vi "extract reports.vi"() -> ()   [LabVIEW 2013]
panel:
  out "error out":errorcluster
  in  "Op":T1(ring)
  out "text":string[](array[string])
  in  "error in":errorcluster
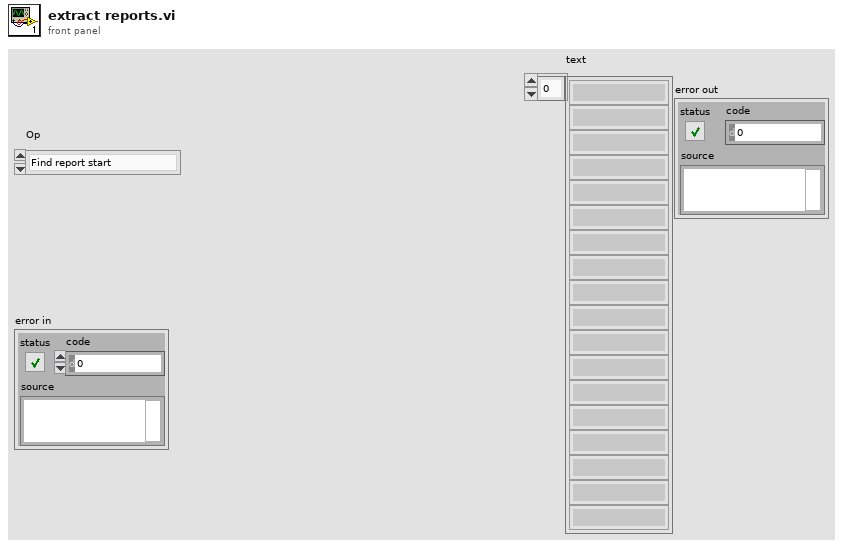
[diagram p1: front panel]
types:
  T1 = enum16{"Find report start", "Collect report body", "Find report end"}
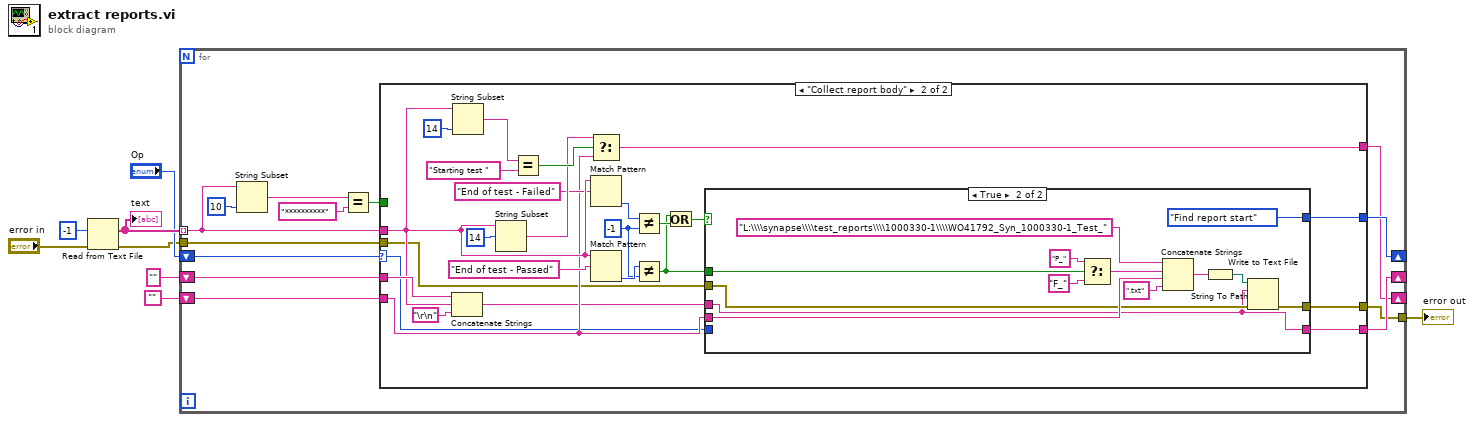
[diagram p0: block diagram]
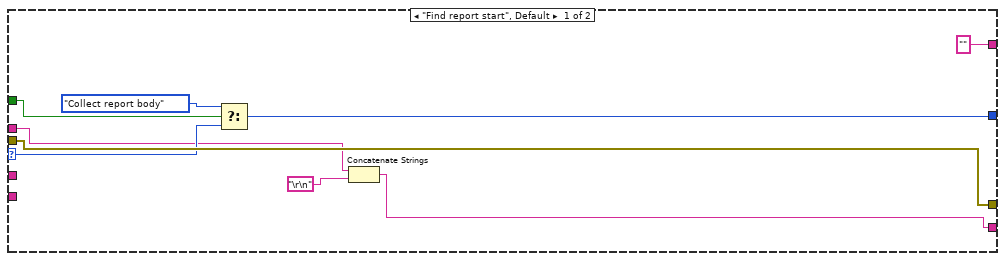
[diagram p2: hidden frame]
diagram:
  n1 = Read from Text File(count=-1, error in="error in") -> (text=w6:string[], error out=w2:errorcluster)  [unwired: 2 in, 2 out]
  "text" <- w6
  n2 = for {
    tunnel: w6 -> [w17] mode=indexing
    shift-right: [w14] -> _
    shift-left: "" -> [w16]
    shift-right: [w13] -> _
    shift-left: "Op" -> [w15]
    shift-right: [w11] -> _
    shift-left: "" -> [w12]
    tunnel: w2 -> [w10]
    tunnel: [w9] -> w1
    n3 = String Subset(string=w17, length (rest)=10 ("length (rest)")) -> (substring=w20:string)  [unwired: 1 in]
    n4 = Equal?(x=w20, y="**********") -> (x = y?=w18:bool)
    n5 = case shown="\"Collect report body\"" w15 {
      selector: w15 -> [w27 w34]
      tunnel: w18 -> [w29 _]
      tunnel: w17 -> [w24 w46]
      tunnel: w16 -> [_ w55]
      tunnel: [w22 w31] -> w14
      tunnel: [w26 w33] -> w13
      tunnel: w12 -> [_ w38]
      tunnel: ["" w48] -> w11
      tunnel: w10 -> [w30 w36]
      tunnel: [w30 w35] -> w9
      frame "Find report start", Default {
        n6 = Select(t=T1."Collect report body" ("Op"), s=w29, f=w27) -> (s? t:f=w26:T1)
        n7 = Concatenate Strings(w24, "\r\n") -> (w22:string)
      }
      frame "Collect report body" {
        w42 = -1 ("y")
        n8 = Concatenate Strings(w55, w46, "\r\n") -> (w37:string)
        n9 = String Subset(string=w46, length (rest)=14 ("length (rest)")) -> (substring=w51:string)  [unwired: 1 in]
        n10 = String Subset(string=w46, offset (0)=14 ("length (rest)")) -> (substring=w49:string)  [unwired: 1 in]
        n11 = Equal?(x=w51, y="Starting test ") -> (x = y?=w52:bool)
        n12 = Select(t=w49, s=w52, f=w38) -> (s? t:f=w48:string)
        n13 = Match Pattern(string=w46, regular expression="End of test - Failed") -> (offset past match=w43:i32)  [unwired: 1 in, 3 out]
        n14 = Match Pattern(string=w46, regular expression="End of test - Passed") -> (offset past match=w44:i32)  [unwired: 1 in, 3 out]
        n15 = Not Equal?(x=w43, y=w42) -> (x != y?=w41:bool)
        n16 = Not Equal?(x=w44, y=w42) -> (x != y?=w39:bool)
        n17 = Or(x=w39, y=w41) -> (x .or. y?=w40:bool)
        n18 = case shown="True" w40 {
          tunnel: w39 -> [_ w71]
          tunnel: w38 -> [_ w66]
          tunnel: w37 -> [w56 w59]
          tunnel: w36 -> [w57 w62]
          tunnel: [w57 w61] -> w35
          tunnel: w34 -> [w58 _]
          tunnel: [w58 T1."Find report start" ("Op")] -> w33
          tunnel: [w56 w59] -> w31
          frame False {
          }
          frame True {
            n19 = Select(t="P_", s=w71, f="F_") -> (s? t:f=w67:string)
            n20 = Concatenate Strings("L:\\\\synapse\\\\test_reports\\\\1000330-1\\\\WO41792_Syn_1000330-1_Test_", w67, w66, ".txt" ("string")) -> (w64:string)
            n21 = String To Path(string=w64) -> (path=w63:path)
            n22 = Write to Text File(file (use dialog)=w63, text=w59, error in=w62) -> (error out=w61:errorcluster)  [unwired: 1 in, 2 out]
          }
        }
      }
    }
  }
  "error out" <- w1
